vi "Magnet_Pulse Magnet.vi"(8 "error in (no error)":errorcluster, 10 "seconds to pulse (6)":dbl[unit]=6.0, 11 "VISA resource name":refnum<visa-resource-name>) -> (0 "error out":errorcluster, 3 "VISA resource name out":refnum<visa-resource-name>)   [LabVIEW 2010]
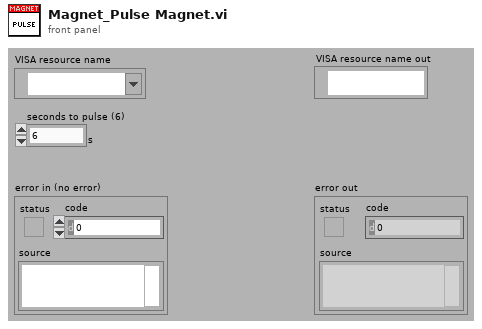
[diagram p1: front panel]
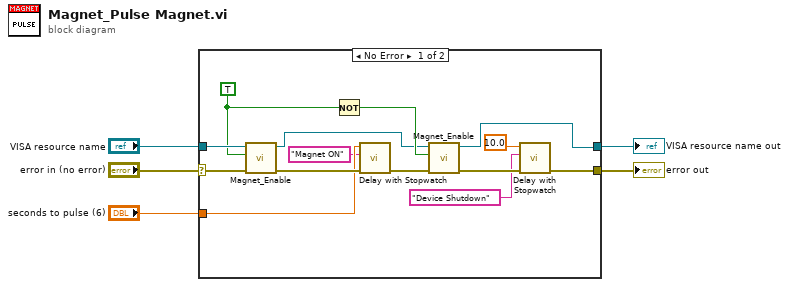
[diagram p0: block diagram]
diagram:
  n1 = case shown="No Error" "error in (no error)" {
    selector: "error in (no error)" -> [w19 w20]
    tunnel: "VISA resource name" -> [w18 w21]
    tunnel: "seconds to pulse (6)" -> [w12 _]
    tunnel: [w8 w20] -> w2
    tunnel: [w10 w21] -> w1
    frame No Error {
      w17 = TRUE ("Enable? (T)")
      n2 = call "Magnet_Enable.vi"("error in (no error)"=w19, "Enable? (T)"=w17, "VISA resource name"=w18) -> ("error out"=w15:errorcluster, "VISA resource name out"=w13:refnum<visa-resource-name>)  [unwired: 7 in]
      n3 = Not(x=w17) -> (.not. x?=w16:bool)
      n4 = call "Delay with Stopwatch.vi"("error in"=w15, "window title"="Magnet ON", "delay"=w12) -> ("error out"=w14:errorcluster)  [unwired: 4 in]
      n5 = call "Magnet_Enable.vi"("error in (no error)"=w14, "Enable? (T)"=w16, "VISA resource name"=w13) -> ("error out"=w9:errorcluster, "VISA resource name out"=w10:refnum<visa-resource-name>)  [unwired: 7 in]
      n6 = call "Delay with Stopwatch.vi"("error in"=w9, "window title"="Device Shutdown", "delay"=dbl[unit] 10.0) -> ("error out"=w8:errorcluster)  [unwired: 4 in]
    }
    frame Error {
    }
  }
  "error out" <- w2
  "VISA resource name out" <- w1
